vi "variableneditor.vi"() -> ()   [LabVIEW 2010]
panel:
  in  "Stopp":bool
  out "gespeicherte Namen":string[](array[string])
  in  "Namen speichern":bool
  in  "neue Namen":string[](array[string])=["Mod1/DIO0", "Mod1/DIO1", "Mod1/DIO2", "Mod4/AI0", "Mod4/AI1", "Mod4/AI2", "Mod5/AI0", "Mod5/AI1", "Mod5/AI2"]
  out "Variablennamen":string[](array[string])=["Mod1/DIO0", "Mod1/DIO1", "Mod1/DIO2", "Mod4/AI0", "Mod4/AI1", "Mod4/AI2", "Mod5/AI0", "Mod5/AI1", "Mod5/AI2"]
  out "Hardware-Schnittstellen":string[](array[string])=["Mod1/DIO0", "Mod1/DIO1", "Mod1/DIO2", "Mod4/AI0", "Mod4/AI1", "Mod4/AI2", "Mod5/AI0", "Mod5/AI1", "Mod5/AI2"]
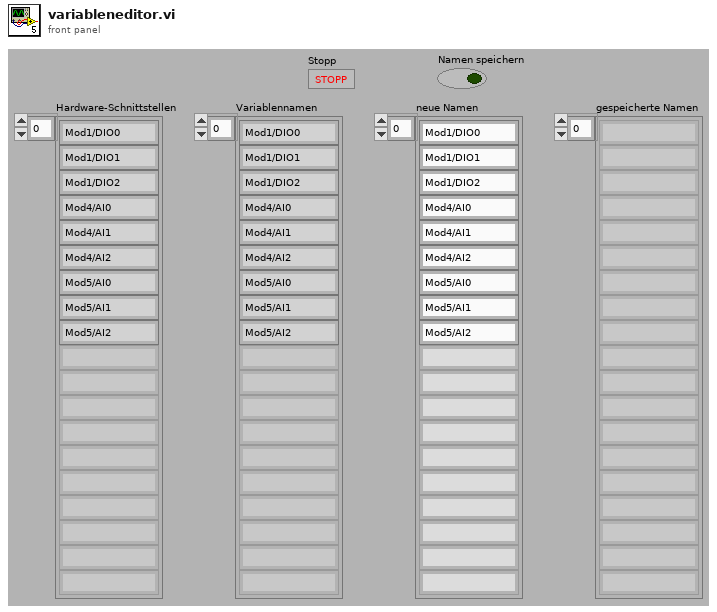
[diagram p1: front panel]
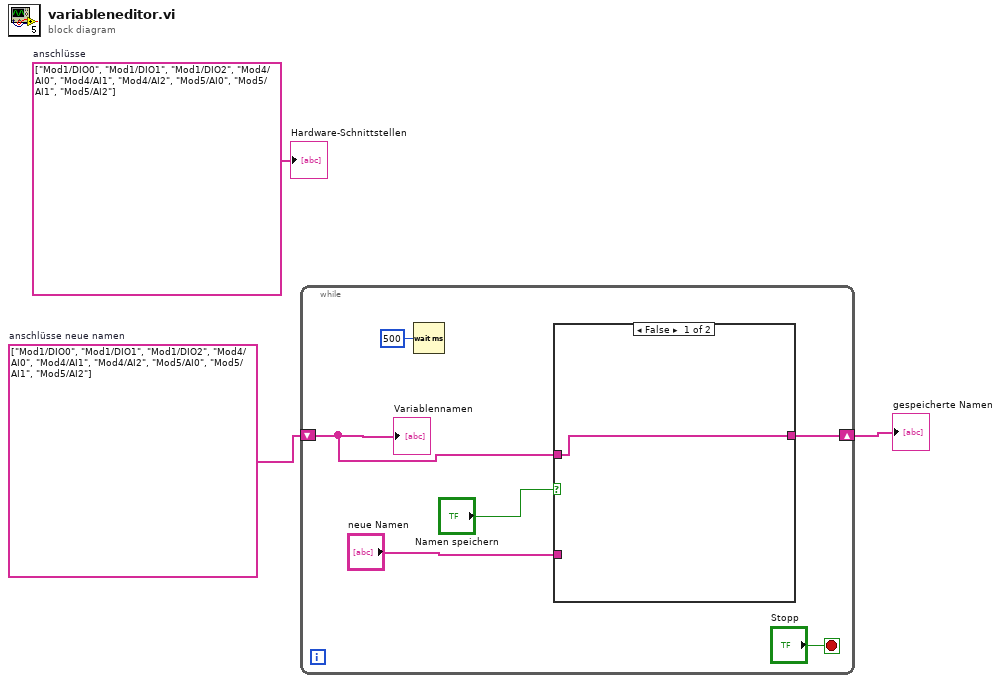
[diagram p0: block diagram]
diagram:
  w2 = string[] ["Mod1/DIO0", "Mod1/DIO1", "Mod1/DIO2", "Mod4/AI0", "Mod4/AI1", "Mod4/AI2", "Mod5/AI0", "Mod5/AI1", "Mod5/AI2"]  # anschlüsse neue namen
  w3 = string[] ["Mod1/DIO0", "Mod1/DIO1", "Mod1/DIO2", "Mod4/AI0", "Mod4/AI1", "Mod4/AI2", "Mod5/AI0", "Mod5/AI1", "Mod5/AI2"]  # anschlüsse
  n1 = while {
    shift-right: [w6] -> w1
    shift-left: w2 -> [w9]
    stop <- "Stopp" stop-if-true
    n2 = Wait (ms)(milliseconds to wait=u32 500 ("Zu wartende ms")) -> ()  [unwired: 1 out]
    n3 = case shown="False" "Namen speichern" {
      tunnel: w9 -> [w10 _]
      tunnel: "neue Namen" -> [_ w11]
      tunnel: [w10 w11] -> w6
      frame False {
      }
      frame True {
      }
    }
    "Variablennamen" <- w9
  }
  "gespeicherte Namen" <- w1
  "Hardware-Schnittstellen" <- w3
